vi "Z Space Adaptation_v1.vi"(6 "deform array":dbl[](array[numeric])=[1.0, 1.0, 1.0, 0.0, 0.0, 0.0, 0.0, 0.0, 0.0], 8 "EyeCenter":dbl[](array[numeric])=[0.0, 10.0], 9 "input (x,y)":dbl[](array[numeric]), 10 "z0":dbl=-2.0, 11 "input z":dbl) -> (3 "z cmd":dbl)   [LabVIEW 2010]
doc: "This VI takes in input (x,y), center z coordinate z0, xy coordinate of eye center, and deformation array to calculate the deformed z coordinate as follows:\n[x',y']' = [x,y]' - EyeCenter;\nz'=z-z0;\nz\"= rc*z' - ra*x'*theta_y + rb*y'*theta_x + z_offset + z0"
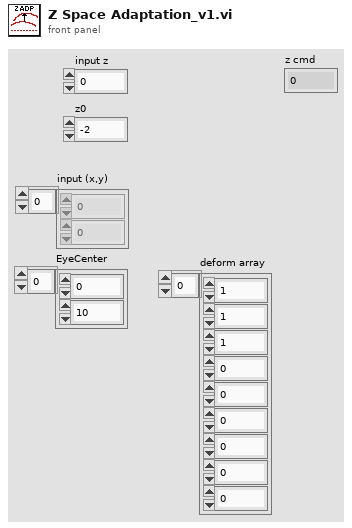
[diagram p1: front panel]
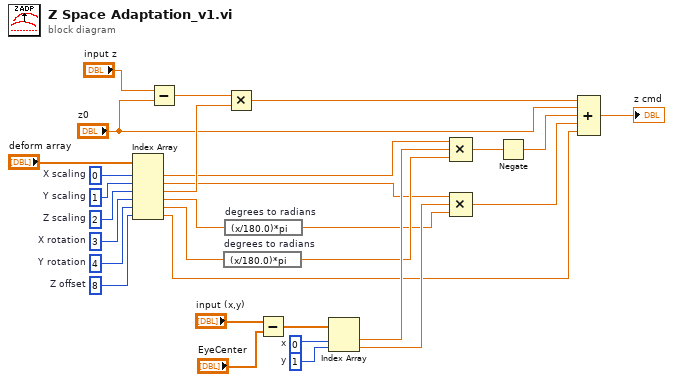
[diagram p0: block diagram]
diagram:
  w16 = 1  # y
  w17 = 0  # x
  w24 = 8  # Z offset
  w25 = 4  # Y rotation
  w26 = 3  # X rotation
  w27 = 2  # Z scaling
  w28 = 1  # Y scaling
  w29 = 0  # X scaling
  n1 = Index Array(array="deform array", index #1=w29, index #2=w28, index #3=w27, index #4=w26, index #5=w25, index #6=w24) -> (element #1=w13:dbl, element #2=w10:dbl, element #3=w20:dbl, element #4=w15:dbl, element #5=w14:dbl, element #6=w4:dbl)
  n2 = Subtract(x="input z", y="z0") -> (x-y=w19:dbl)
  n3 = expression code="(x/180.0)*pi" "degrees to radians"(w14) -> (w11:dbl)
  n4 = expression code="(x/180.0)*pi" "degrees to radians"(w15) -> (w8:dbl)
  n5 = Multiply(x=w19, y=w20) -> (x*y=w3:dbl)
  n6 = Subtract(x="input (x,y)", y="EyeCenter") -> (x-y=w18:dbl[])
  n7 = Index Array(array=w18, index #1=w17, index #2=w16) -> (element #1=w12:dbl, element #2=w9:dbl)
  n8 = Compound Arithmetic op=MULTIPLY(w13, w12, w11) -> (w7:dbl)
  n9 = Compound Arithmetic op=MULTIPLY(w10, w9, w8) -> (w5:dbl)
  n10 = Negate(x=w7) -> (-x=w6:dbl)
  n11 = Compound Arithmetic op=ADD(w3, "z0", w6, w5, w4) -> (→"z cmd":dbl)
